vi "Multi Detected.vi"(8 "error in (no error)":errorcluster, 10 "Targets in":T1 {"Filtered Targets"."IP Mode" items=["Static"=1, "DHCP/Link-Local"=2, "Link-Local Only"=4, "DHCP Only"=8]}, 11 "Ctl Refs in":T4) -> (0 "error out":errorcluster, 2 "Targets out":T1 {"Filtered Targets"."IP Mode" items=["Static"=1, "DHCP/Link-Local"=2, "Link-Local Only"=4, "DHCP Only"=8]}, 3 "Ctl Refs out":T4)   [LabVIEW 2013]
uses:
  Controls/Refs.ctl
  Controls/Button Refs.ctl
  Controls/Tab Ctl Refs.ctl
  types/TabStateType.ctl
  Controls/Indicator Refs.ctl
  Controls/Slider Refs.ctl
  Controls/Control Refs.ctl
  Controls/Targets.ctl
  Controls/Detected.ctl
  types/MAX Sys Cfg Target Information.ctl
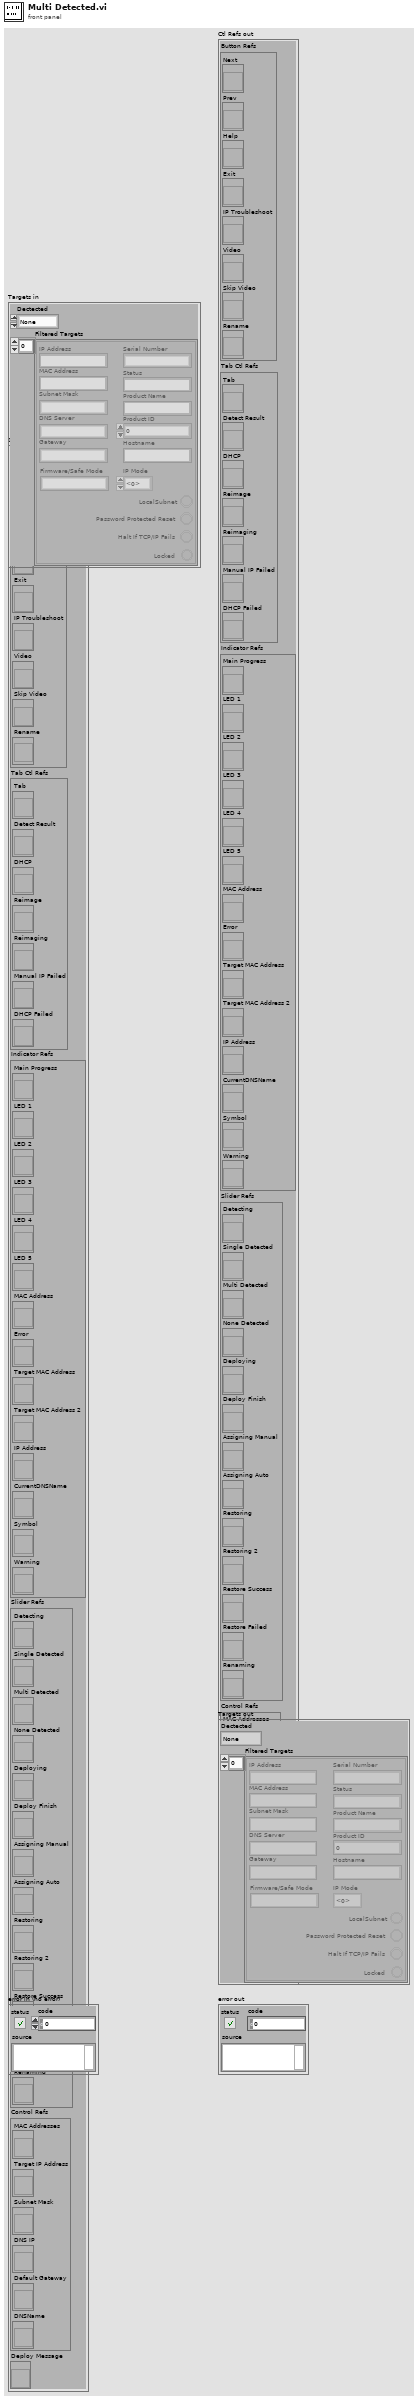
[diagram p1: front panel]
types:
  T1 = typedef "Targets.ctl" = cluster{"Dectected":T2, "Filtered Targets":T3[]}
  T2 = typedef "Detected.ctl" = enum16{"None", "Failed", "Single", "Multi"}
  T3 = typedef "MAX Sys Cfg Target Information.ctl" = cluster{"MAC Address":string, "IP Address":string, "Status":string, "Product Name":string, "Hostname":string, "Firmware/Safe Mode":string, "Subnet Mask":string, "Gateway":string, "DNS Server":string, "Serial Number":string, "Product ID":u32, "Locked ":bool, "LocalSubnet":bool, "Halt If TCP/IP Fails":bool, "Password Protected Reset":bool, "IP Mode":i32}
  T4 = typedef "Refs.ctl" = cluster{"Button Refs":T5, "Tab Ctl Refs":T6, "Indicator Refs":T7, "Slider Refs":T8, "Control Refs":T9, "Deploy Message":refnum<vi>}
  T5 = typedef "Button Refs.ctl" = cluster{"Next":refnum<vi>, "Prev":refnum<vi>, "Help":refnum<vi>, "Exit":refnum<vi>, "IP Troubleshoot":refnum<vi>, "Video":refnum<vi>, "Skip Video":refnum<vi>, "Rename":refnum<vi>}
  T6 = typedef "Tab Ctl Refs.ctl" = cluster{"Tab":refnum<vi>, "Detect Result":refnum<vi>, "DHCP":refnum<vi>, "Reimage":refnum<vi>, "Reimaging":refnum<vi>, "Manual IP Failed":refnum<vi>, "DHCP Failed":refnum<vi>}
  T7 = typedef "Indicator Refs.ctl" = cluster{"Main Progress":refnum<vi>, "LED 1":refnum<vi>, "LED 2":refnum<vi>, "LED 3":refnum<vi>, "LED 4":refnum<vi>, "LED 5":refnum<vi>, "MAC Address":refnum<vi>, "Error":refnum<vi>, "Target MAC Address":refnum<vi>, "Target MAC Address 2":refnum<vi>, "IP Address":refnum<vi>, "CurrentDNSName":refnum<vi>, "Symbol":refnum<vi>, "Warning":refnum<vi>}
  T8 = typedef "Slider Refs.ctl" = cluster{"Detecting":refnum<vi>, "Single Detected":refnum<vi>, "Multi Detected":refnum<vi>, "None Detected":refnum<vi>, "Deploying":refnum<vi>, "Deploy Finish":refnum<vi>, "Assigning Manual":refnum<vi>, "Assigning Auto":refnum<vi>, "Restoring":refnum<vi>, "Restoring 2":refnum<vi>, "Restore Success":refnum<vi>, "Restore Failed":refnum<vi>, "Renaming":refnum<vi>}
  T9 = typedef "Control Refs.ctl" = cluster{"MAC Addresses":refnum<vi>, "Target IP Address":refnum<vi>, "Subnet Mask":refnum<vi>, "DNS IP":refnum<vi>, "Default Gateway":refnum<vi>, "DNSName":refnum<vi>}
  T10 = enum32{"Welcome", "Instructions", "Detect", "Run Detection", "Detect Result", "Deploy", "Run Deployment", "Connect Verify", "Success"}
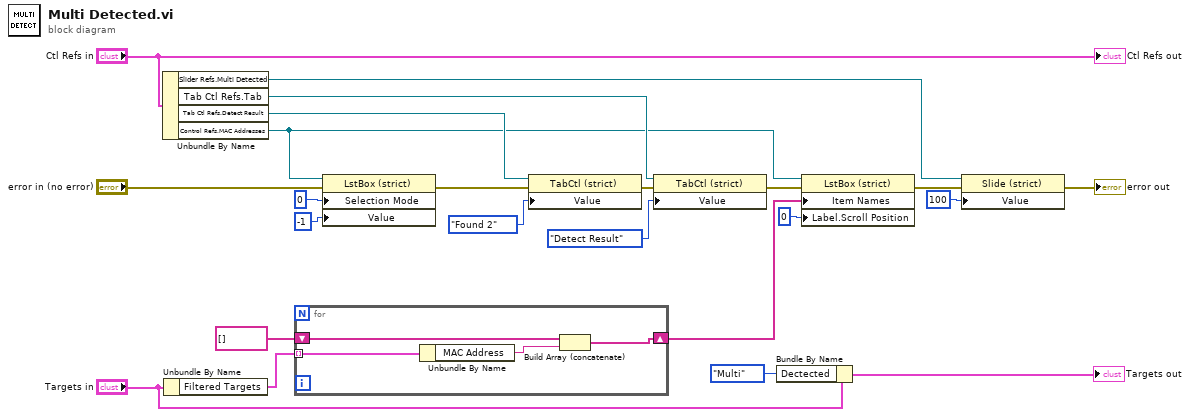
[diagram p0: block diagram]
diagram:
  n1 = Unbundle By Name("Ctl Refs in") -> ("Slider Refs.Multi Detected"=w2:refnum<vi>, "Tab Ctl Refs.Tab"=w5:refnum<vi>, "Tab Ctl Refs.Detect Result"=w6:refnum<vi>, "Control Refs.MAC Addresses"=w4:refnum<vi>)
  n2 = Unbundle By Name("Targets in") -> ("Filtered Targets"=w8:T3[])
  n3 = for {
    tunnel: w8 -> [w27] mode=indexing
    shift-right: [w26] -> w16
    shift-left: string[] [] -> [w25]
    n4 = Unbundle By Name(w27) -> ("MAC Address"=w24:string)
    n5 = Build Array (concatenate)(w25, w24) -> (w26:string[])
  }
  n6 = property on="Property Node" class="LstBox (strict)"(reference=w4, error in="error in (no error)", "Selection Mode"=0, "Value"=-1 ("Serial Numbers:")) -> (error out=w12:errorcluster)  [unwired: 1 out]
  n7 = property on="Property Node" class="TabCtl (strict)"(reference=w6, error in=w12, "Value"=enum32{"Found 0", "Found 1", "Found 2"}."Found 2" ("Detect Result Tabs")) -> (error out=w13:errorcluster)  [unwired: 1 out]
  n8 = property on="Property Node" class="TabCtl (strict)"(reference=w5, error in=w13, "Value"=T10."Detect Result" ("Tab Control")) -> (error out=w11:errorcluster)  [unwired: 1 out]
  n9 = Bundle By Name(cluster="Targets in", "Dectected"=Detected."Multi") -> (→"Targets out":T1)
  n10 = property on="Property Node" class="LstBox (strict)"(reference=w4, error in=w11, "Item Names"=w16, "Label.Scroll Position"=u32 0) -> (error out=w3:errorcluster)  [unwired: 1 out]
  n11 = property on="Property Node" class="Slide (strict)"(reference=w2, error in=w3, "Value"=i8 100 ("Slide 6")) -> (error out=→"error out":errorcluster)  [unwired: 1 out]
  "Ctl Refs out" <- "Ctl Refs in"
